vi "Max-Min.vi"(0 "Color Plane (Color Plane Extraction 1)":i32(ring)=6 items=["Red", "Green", "Blue", "Hue", "Saturation", "Luminance", "Value", "Intensity"], 1 "Operator (Lookup Table 1)":T2(ring)=enum."Power X", 2 "X Value (Lookup Table 1)":sgl=1.5) -> (20 "Results (Quantify 1)":sgl[][](array[numeric]) format="%.2f", 27 "error out":errorcluster)   [LabVIEW 2009]
uses:
  <vilib>/vision/Image Controls.llb/IMAQ Image.ctl
  <vilib>/vision/NI_Vision_Development_Module.lvlib
panel:
  in  "error in (no error)":errorcluster
  in  "Image Src":T1
  out "Number of ramp regions":i32
  in  "Tolerance":sgl=50.0
  out "Array":i32[](array[numeric])
  out "Standard (?) deviation of image":sgl
  in  "stop":bool
  in  "ROI index":i32(knob) scale=1.0..9.0
  out "Max-Min Array":sgl[](array[numeric])
  out "Image Out":T1(plugin-control)
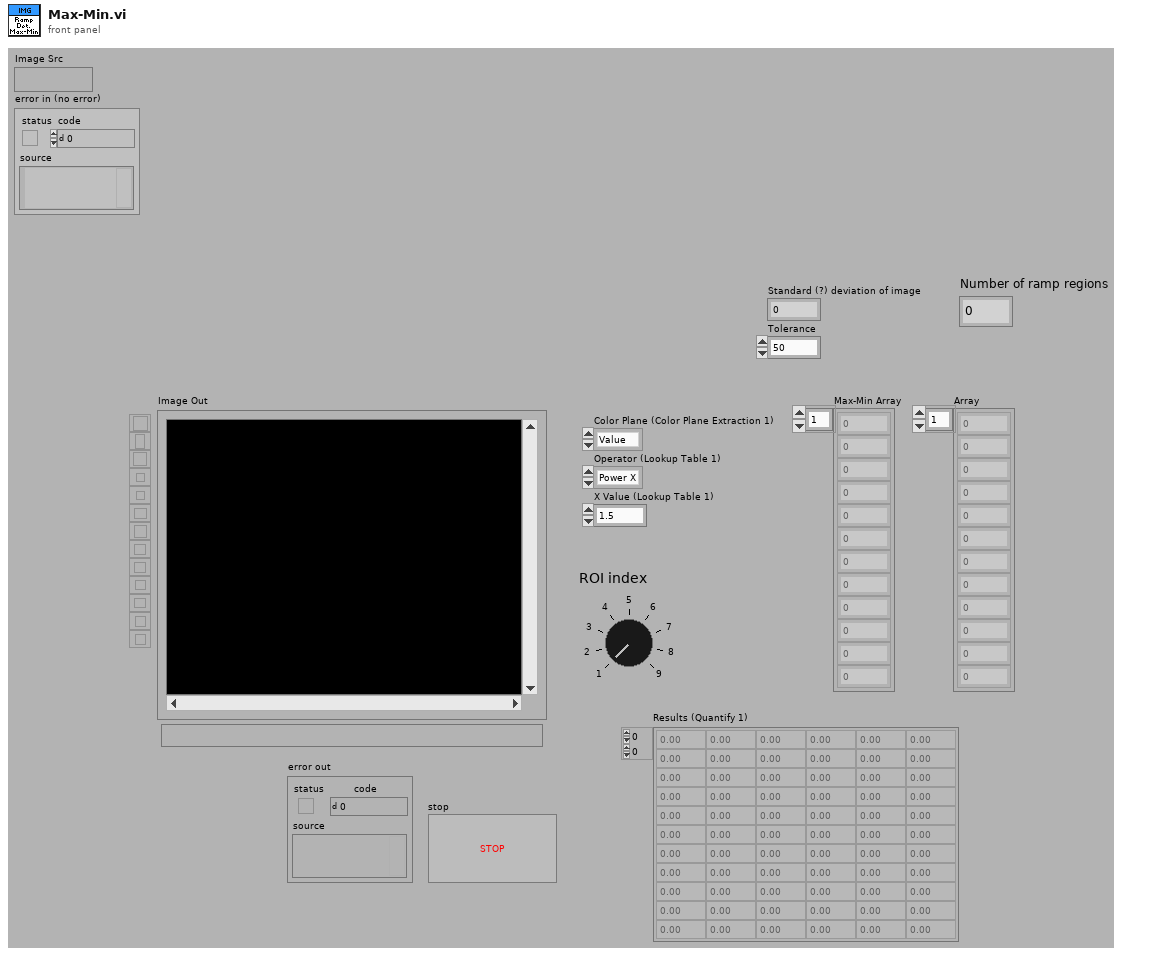
[diagram p1: front panel]
types:
  T1 = typedef "IMAQ Image.ctl" = refnum<image>
  T2 = enum32{"Linear", "Log", "Exp", "Square", "Square root", "Power X", "Power 1/X"}
  T3 = cluster{"Global Rectangle":i32[], "Contours":cluster{"ID":enum32{"External", "Internal"}, "Type":u32, "Coordinates":i32[]}[]}[]
  T4 = cluster{"Global Rectangle":i32[], "Contours":cluster{"ID":enum32{"External", "Internal"}, "Type":u32, "Coordinates":i32[]}[]}
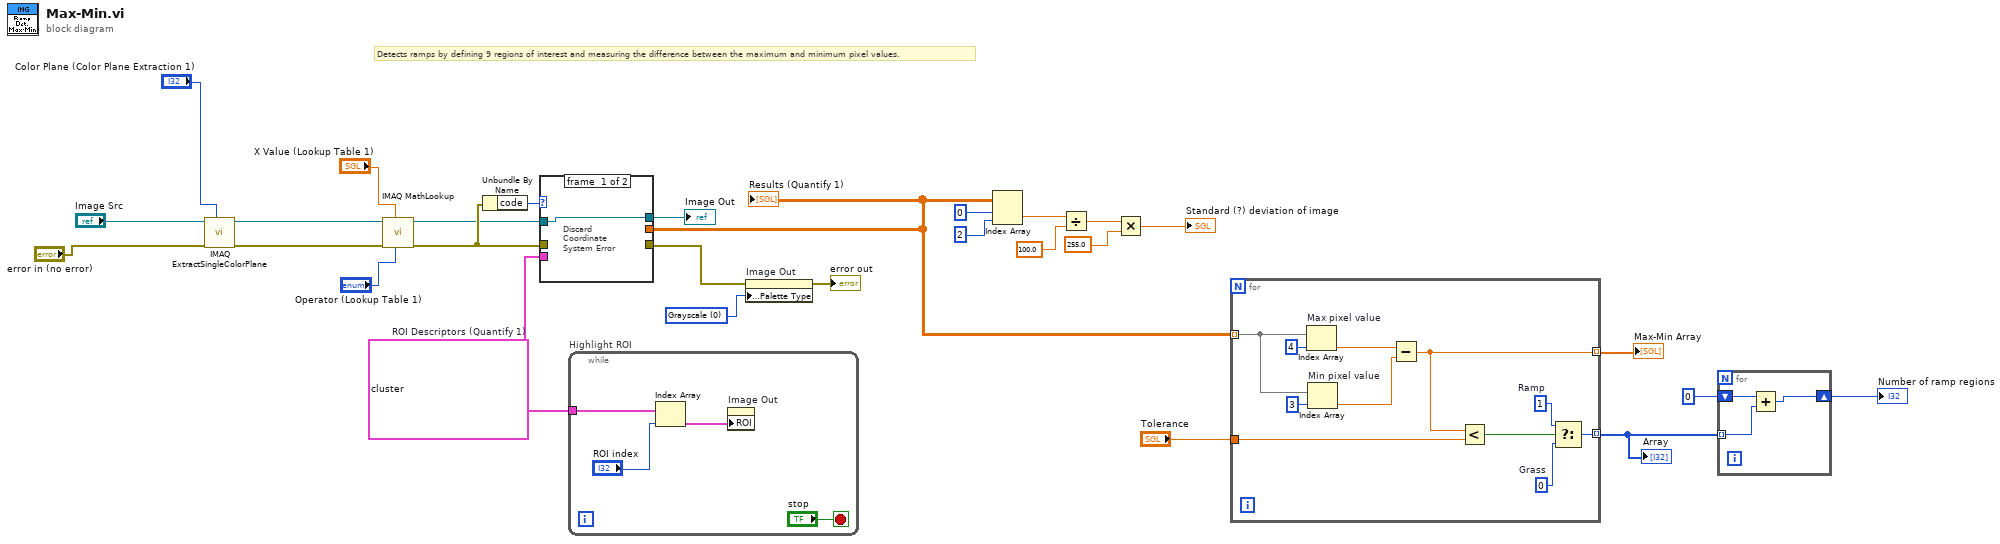
[diagram p0: block diagram]
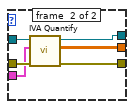
[diagram p2: hidden frame]
diagram:
  w15 = T3 [{"Global Rectangle"=[0, 0, 160, 120], "Contours"=[{"ID"=enum."External", "Type"=3, "Coordinates"=[0, 0, 160, 120]}]}, {"Global Rectangle"=[18, 13, 28, 23], "Contours"=[{"ID"=enum."External", "Type"=3, "Coordinates"=[18, 13, 28, 23]}]}, {"Global Rectangle"=[77, 13, 87, 23], "Contours"=[{"ID"=enum."External", "Type"=3, "Coordinates"=[77, 13, 87, 23]}]}, {"Global Rectangle"=[135, 12, 145, 23], "Contours"=[{"ID"=enum."External", "Type"=3, "Coordinates"=[135, 12, 145, 23]}]}, {"Global Rectangle"=[18, 53, 28, 64], "Contours"=[{"ID"=enum."External", "Type"=3, "Coordinates"=[18, 53, 28, 64]}]}, {"Global Rectangle"=[77, 53, 87, 64], "Contours"=[{"ID"=enum."External", "Type"=3, "Coordinates"=[77, 53, 87, 64]}]}, {"Global Rectangle"=[137, 54, 146, 64], "Contours"=[{"ID"=enum."External", "Type"=3, "Coordinates"=[137, 54, 146, 64]}]}, {"Global Rectangle"=[18, 92, 28, 102], "Contours"=[{"ID"=enum."External", "Type"=3, "Coordinates"=[18, 92, 28, 102]}]}, {"Global Rectangle"=[77, 90, 87, 100], "Contours"=[{"ID"=enum."External", "Type"=3, "Coordinates"=[77, 90, 87, 100]}]}, {"Global Rectangle"=[136, 88, 146, 99], "Contours"=[{"ID"=enum."External", "Type"=3, "Coordinates"=[136, 88, 146, 99]}]}]  # ROI Descriptors (Quantify 1)
  w18 = u32 0 items=["Grayscale", "Binary", "Gradient", "Rainbow", "Temperature", "User Defined"] ("Palette")
  # "Detects ramps by defining 9 regions of interest and measuring the difference between the maximum and minimum pixel values."
  n1 = call "IMAQ ExtractSingleColorPlane"("Color Plane"="Color Plane (Color Plane Extraction 1)", "error in (no error)"="error in (no error)", "Image Src"="Image Src") -> ("error out"=w27:errorcluster, "Image Dst Out"=w24:T1)  [unwired: 1 in, 6 out]
  n2 = call "IMAQ MathLookup"("Operator"="Operator (Lookup Table 1)", "X Value"="X Value (Lookup Table 1)", "error in (no error)"=w27, "Image Src"=w24) -> ("error out"=w23:errorcluster, "Image Dst Out"=w22:T1)  [unwired: 3 in, 3 out]
  n3 = Unbundle By Name(w23) -> ("code"=w20:i32)
  n4 = case shown="Default" w20 {
    tunnel: [_ w35] -> w14
    tunnel: w22 -> [w29 w34]
    tunnel: w23 -> [_ w33]
    tunnel: [w29 w32] -> w19
    tunnel: [_ w31] -> w21
    tunnel: w15 -> [_ w30]
    frame #0 {
      # "Discard\nCoordinate\nSystem Error"
    }
    frame #1 {
      n5 = call <vilib>:"IVA Quantify.vi"("error in (no error)"=w33, "ROI Descriptors"=w30, "Image"=w34) -> ("error out"=w31:errorcluster, "Results"=w35:sgl[][], "Image Out"=w32:T1)  [unwired: 6 out]
    }
  }
  "Results (Quantify 1)" <- w14
  "Image Out" <- w19
  n6 = while "Highlight ROI" {
    tunnel: w15 -> [w39]
    stop <- "stop" stop-if-true
    n7 = Index Array(array=w39, index="ROI index") -> (element=w37:T4)
    n8 = property on="Image Out" class="ImageControl"("ROI"=w37) -> ()  [unwired: 2 in, 2 out]
  }
  n9 = property on="Image Out" class="ImageControl"(error in=w21, "Palette:Palette Type"=w18) -> (error out=→"error out":errorcluster)  [unwired: 1 in, 1 out]
  n10 = Index Array(array=w14, index (row)=0, index (col)=2 ("disabled index (col)")) -> (element=w11:sgl)
  n11 = Divide(x=w11, y=sgl 100.0) -> (x/y=w9:sgl)
  n12 = Multiply(x=w9, y=sgl 255.0) -> (x*y=→"Standard (?) deviation of image":sgl)
  n13 = for {
    tunnel: w14 -> [w42] mode=indexing
    tunnel: [w41] -> w16 mode=indexing
    tunnel: "Tolerance" -> [w46]
    tunnel: [w43] -> w4 mode=indexing
    w44 = 0  # Grass
    w45 = 1  # Ramp
    n14 = Index Array "Max pixel value"(array=w42, index=4) -> (element=w48:sgl)
    n15 = Index Array "Min pixel value"(array=w42, index=3) -> (element=w47:sgl)
    n16 = Subtract(x=w48, y=w47) -> (x-y=w41:sgl)
    n17 = Less?(x=w41, y=w46) -> (x < y?=w40:bool)
    n18 = Select(t=w45, s=w40, f=w44) -> (s? t:f=w43:i32)
  }
  "Max-Min Array" <- w16
  "Array" <- w4
  n19 = for {
    shift-right: [w51] -> w3
    shift-left: 0 ("s? t:f") -> [w53]
    tunnel: w4 -> [w52] mode=indexing
    n20 = Add(x=w53, y=w52) -> (x+y=w51:i32)
  }
  "Number of ramp regions" <- w3
